vi "Read MUS EventH.vi"(11 "MUS_Data_in":u8[](array[numeric])) -> (0 "CAHN":u8, 1 "Even_No":u8, 2 "Last flag?":bool, 3 "Data_Remaining":u8[](array[numeric]))   [LabVIEW 2014]
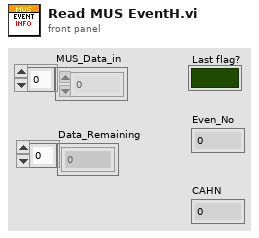
[diagram p1: front panel]
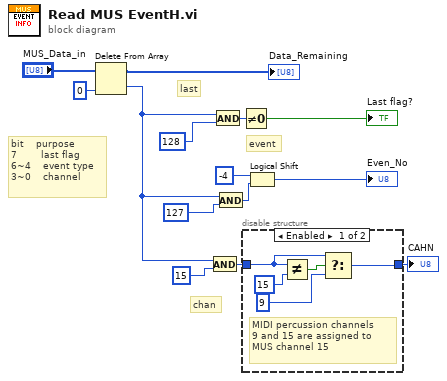
[diagram p0: block diagram]
diagram:
  # "bit    purpose\n7        last flag\n6~4    event type\n3~0    channel"
  # "event"
  # "chan"
  # "last"
  n1 = Delete From Array(array="MUS_Data_in", index=0) -> (deleted portion=w7:u8, array with subset deleted=→"Data_Remaining":u8[])  [unwired: 1 in]
  n2 = And(x=w7, y=u8 15) -> (x .and. y?=w13:u8)
  n3 = And(x=w7, y=u8 128) -> (x .and. y?=w9:u8)
  n4 = And(x=w7, y=u8 127) -> (x .and. y?=w3:u8)
  n5 = Not Equal To 0?(x=w9) -> (x != 0?=→"Last flag?":bool)
  n6 = disable-structure shown="Enabled" {
    disable-tunnel: [w19 w20] -> w14
    disable-tunnel: w13 -> [w16 w20]
    frame Enabled {
      # "MIDI percussion channels \n9 and 15 are assigned to \nMUS channel 15"
      n7 = Not Equal?(x=w16, y=u8 15) -> (x != y?=w15:bool)
      n8 = Select(t=w16, s=w15, f=u8 9) -> (s? t:f=w19:u8)
    }
    frame Disabled {
    }
  }
  "CAHN" <- w14
  n9 = Logical Shift(y=i16 -4, x=w3) -> (x << y=→"Even_No":u8)
